vi "JSON ISO8601 to Timestamp.vi"(11 "ISO 8601 Date Time":string) -> (3 "Local Time Stamp":timestamp format="%<%Y-%m-%dT%H:%M:%S%6u>T")   [LabVIEW 2019, in "labview_json.lvlib"]
uses:
  labview_json.lvlib
  <vilib>/regexp/Match Regular Expression.xnode
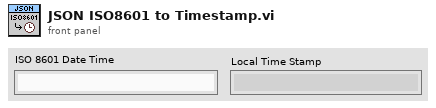
[diagram p1: front panel]
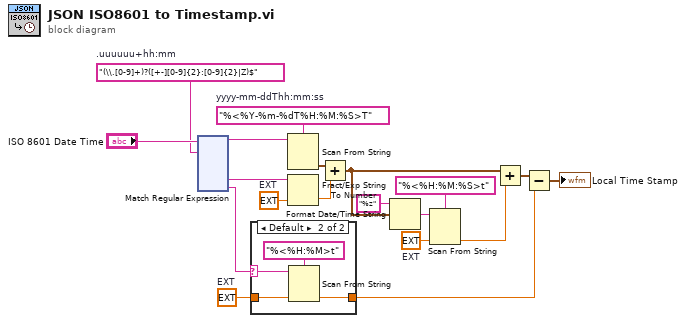
[diagram p0: block diagram]
diagram:
  w2 = ext 0.0  # EXT
  w10 = ext 0.0  # EXT
  w15 = "%<%Y-%m-%dT%H:%M:%S>T"  # yyyy-mm-ddThh:mm:ss
  w17 = ext 0.0  # EXT
  w18 = "(\\.[0-9]+)?([+-][0-9]{2}:[0-9]{2}|Z)$"  # .uuuuuu+hh:mm
  n1 = xnode "Match Regular Expression"("input string"="ISO 8601 Date Time", "regular expression"=w18) -> ("before match"=w16:string, "submatch 1"=w3:string, "submatch 2"=w5:string)  [unwired: 4 in, 4 out]
  n2 = case shown="Default" w5 {
    selector: w5 -> [_ w24]
    tunnel: w17 -> [w20 w22]
    tunnel: [w20 w21] -> w14
    frame "", "Z" {
    }
    frame Default {
      n3 = Scan From String(format string="%<%H:%M>t", input string=w24, default 1=w22) -> (output 1=w21:ext)  [unwired: 2 in, 3 out]
    }
  }
  n4 = Scan From String(format string=w15, input string=w16) -> (output 1=w8:timestamp)  [unwired: 3 in, 3 out]
  n5 = Fract/Exp String To Number(string=w3, default (0 dbl)=w2) -> (number=w1:ext)  [unwired: 2 in, 1 out]
  n6 = Add(x=w8, y=w1) -> (x+y=w4:timestamp)
  n7 = Format Date/Time String(time format string (%c)="%z", seconds (now)=w4) -> (date/time string=w11:string)  [unwired: 1 in]
  n8 = Scan From String(format string="%<%H:%M:%S>t", input string=w11, default 1=w10) -> (output 1=w9:ext)  [unwired: 2 in, 3 out]
  n9 = Add(x=w4, y=w9) -> (x+y=w7:timestamp)
  n10 = Subtract(x=w7, y=w14) -> (x-y=→"Local Time Stamp":timestamp)
